vi "PXI-Find DIO Clock Source.vi"(8 "error in (no error)":errorcluster, 10 "DAQmx Device Name":tag="PXI1Slot4", 11 "Sync Task":T1) -> (0 "error out":errorcluster, 3 "Counter Task":T1={"Task name"="Counter", "Task"="", "Dual-channel task?"=FALSE, "Regenerate?"=FALSE, "Clear?"=FALSE})   [LabVIEW 2020]
uses:
  Type Defs/Task Struct.ctl
  PXI Globals.vi
  <vilib>/DAQmx/create/channels.llb/DAQmx Create Channel (CO-Pulse Generation-Ticks).vi
  <vilib>/DAQmx/configure/timing.llb/DAQmx Timing (Implicit).vi
  <vilib>/DAQmx/configure/trigger.llb/DAQmx Start Trigger (Digital Edge).vi
  <resource>/objmgr/daqmx.rc
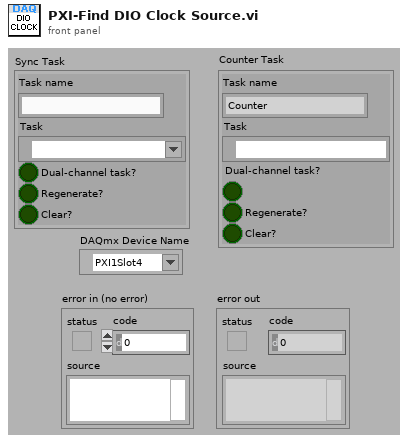
[diagram p1: front panel]
types:
  T1 = typedef "Task Struct.ctl" = cluster{"Task name":string, "Task":refnum<k21>, "Dual-channel task?":bool, "Regenerate?":bool, "Clear?":bool}
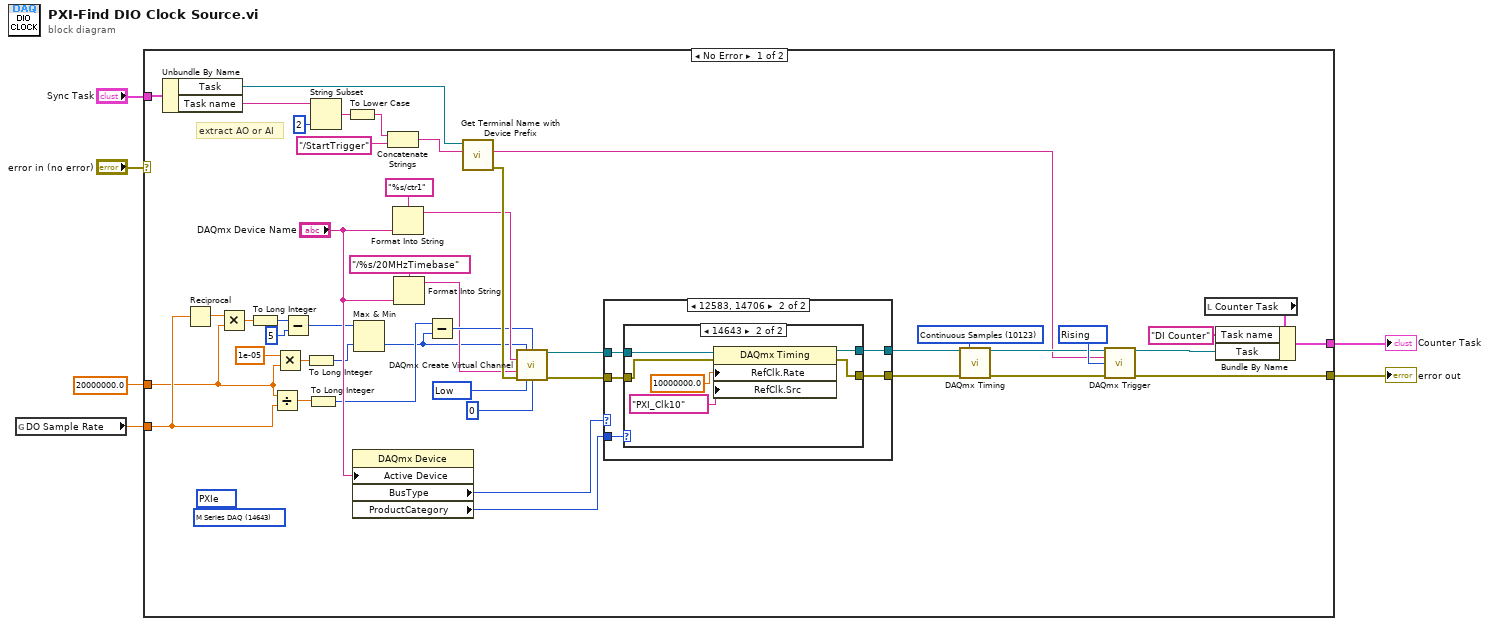
[diagram p0: block diagram]
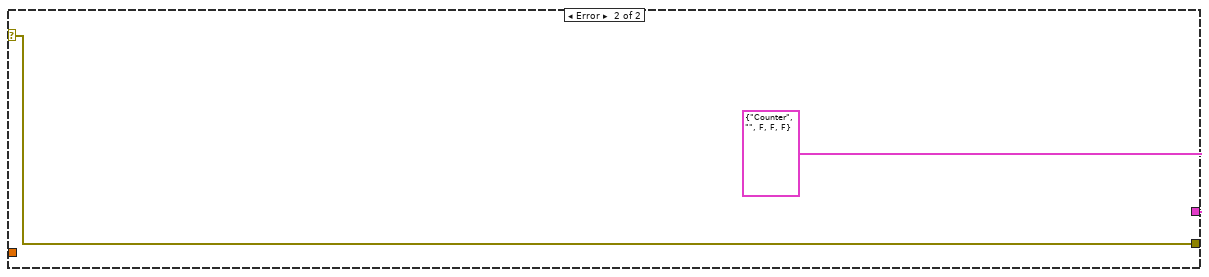
[diagram p4: hidden frame]
diagram:
  n1 = global read "PXI Globals.vi" "DO Sample Rate"() -> (w2:dbl)
  n2 = case shown="No Error" "error in (no error)" {
    selector: "error in (no error)" -> [_ w68]
    tunnel: [w52 w68] -> w6
    tunnel: "Sync Task" -> [w51 _]
    tunnel: [w50 T1 {"Task name"="Counter", "Task"="", "Dual-channel task?"=FALSE, "Regenerate?"=FALSE, "Clear?"=FALSE} ("Counter Task")] -> w5
    tunnel: w2 -> [w16 _]
    tunnel: 20000000.0 ("x") -> [w13 _]
    frame No Error {
      (unwired) 14643 items=["M Series DAQ"=14643, "X Series DAQ"=15858, "E Series DAQ"=14642, "S Series DAQ"=14644, "B Series DAQ"=14662, "SC Series DAQ"=14645, "USB DAQ"=14646, "AO Series"=14647, "Digital I/O"=14648, "TIO Series"=14661, "Dynamic Signal Acquisition"=14649, "Switches"=14650, "CompactDAQ Chassis"=14658, "C Series Module"=14659, "SCXI Module"=14660, "SCC Connector Block"=14704, "SCC Module"=14705, "NI ELVIS"=14755, "Network DAQ"=14829, "SC Express"=15886, "Unknown"=12588] ("ProductCategory")
      (unwired) 14706 items=["PCI"=12582, "PCIe"=13612, "PXI"=12583, "PXIe"=14706, "SCXI"=12584, "SCC"=14707, "PCCard"=12585, "USB"=12586, "CompactDAQ"=14637, "TCP/IP"=14828, "Unknown"=12588, "SwitchBlock"=15870] ("BusType")
      w25 = 10214 items=["High"=10192, "Low"=10214] ("idle state")
      w48 = 10280 items=["Rising"=10280, "Falling"=10171] ("Trigger Edge")
      w49 = 10123 items=["Finite Samples"=10178, "Continuous Samples"=10123] ("sample mode")
      # "extract AO or AI"
      n3 = Unbundle By Name(w51) -> ("Task"=w30:refnum<k21>, "Task name"=w42:string)
      n4 = Reciprocal(x=w16) -> (1/x=w14:dbl)
      n5 = Multiply(x=w14, y=w13) -> (x*y=w15:dbl)
      n6 = To Long Integer(number=w15) -> (32bit integer=w12:i32)
      n7 = Divide(x=w13, y=w16) -> (x/y=w22:dbl)
      n8 = Multiply(x=1e-05, y=w13) -> (x*y=w23:dbl)
      n9 = Subtract(x=w12, y=5) -> (x-y=w10:i32)
      n10 = To Long Integer(number=w23) -> (32bit integer=w9:i32)
      n11 = To Long Integer(number=w22) -> (32bit integer=w8:i32)
      n12 = String Subset(string=w42, length (rest)=2 ("length (rest)")) -> (substring=w41:string)  [unwired: 1 in]
      n13 = To Lower Case(string=w41) -> (all lower case string=w35:string)
      n14 = property class="DAQmx Device"("Active Device"="DAQmx Device Name") -> ("BusType"=w18:i32, "ProductCategory"=w17:i32)  [unwired: 2 in, 2 out]
      n15 = Max & Min(x=w10, y=w9) -> (min(x,y)=w7:i32)  [unwired: 1 out]
      n16 = Concatenate Strings(w35, "/StartTrigger" ("Local Terminal Name")) -> (w44:string)
      n17 = Format Into String(format string="%s/ctr1", "DAQmx Device Name") -> (resulting string=w27:string)  [unwired: 2 in, 1 out]
      n18 = Format Into String(format string="/%s/20MHzTimebase", "DAQmx Device Name") -> (resulting string=w19:string)  [unwired: 2 in, 1 out]
      n19 = Subtract(x=w8, y=w7) -> (x-y=w21:i32)
      n20 = call "Get Terminal Name with Device Prefix.vi"("Local Terminal Name"=w44, "task/channels in"=w30) -> ("error out"=w34:errorcluster, "Terminal Name with Device Prefix"=w36:tag)  [unwired: 7 in, 1 out]
      n21 = call-poly <vilib>:"DAQmx Create Virtual Channel.vi"("high ticks"=w7, "low ticks"=w21, "counter"=w27, "source of ticks"=w19, "error in"=w34, "idle state"=w25, "initial delay"=u32 0) -> ("task out"=w32:refnum<k21>, "error out"=w33:errorcluster)  [unwired: 7 in]
      n22 = case shown="12583, 14706" w18 {
        tunnel: [w54 w59] -> w40
        tunnel: [w53 w58] -> w39
        tunnel: w33 -> [w53 w57]
        tunnel: w32 -> [w54 w56]
        tunnel: w17 -> [_ w55]
        frame 0, Default {
        }
        frame 12583, 14706 {
          n23 = case shown="14643" w55 {
            tunnel: [w61 w67] -> w59
            tunnel: [w60 w66] -> w58
            tunnel: w57 -> [w60 w65]
            tunnel: w56 -> [w61 w64]
            frame 0, Default {
            }
            frame 14643 {
              n24 = property class="DAQmx Timing"(reference=w64, error in=w65, "RefClk.Rate"=10000000.0, "RefClk.Src"=tag "PXI_Clk10") -> (reference out=w67:refnum<k21>, error out=w66:errorcluster)
            }
          }
        }
      }
      n25 = call-poly <vilib>:"DAQmx Timing.vi"("task/channels in"=w40, "sample mode"=w49, "error in"=w39) -> ("task out"=w38:refnum<k21>, "error out"=w37:errorcluster)  [unwired: 11 in]
      n26 = call-poly <vilib>:"DAQmx Trigger.vi"("task/channels in"=w38, "source"=w36, "edge"=w48, "error in"=w37) -> ("task out"=w46:refnum<k21>, "error out"=w52:errorcluster)  [unwired: 10 in]
      n27 = local read "Counter Task"() -> (w31:T1)
      n28 = Bundle By Name(cluster=w31, "Task name"="DI Counter" ("Channel"), "Task"=w46) -> (w50:T1)
    }
    frame Error {
    }
  }
  "error out" <- w6
  "Counter Task" <- w5
